vi "Detect Failed.vi"(8 "error in (no error)":errorcluster, 9 "Software-Only?":bool, 10 "Targets in":T1 {"Filtered Targets"."IP Mode" items=["Static"=1, "DHCP/Link-Local"=2, "Link-Local Only"=4, "DHCP Only"=8]}, 11 "Ctl Refs in":T5) -> (0 "error out":errorcluster, 1 "Enum":T4, 2 "Targets out":T1 {"Filtered Targets"."IP Mode" items=["Static"=1, "DHCP/Link-Local"=2, "Link-Local Only"=4, "DHCP Only"=8]}, 3 "Ctl Refs out":T5)   [LabVIEW 2013]
uses:
  Controls/Refs.ctl
  Controls/Button Refs.ctl
  Controls/Tab Ctl Refs.ctl
  types/TabStateType.ctl
  Controls/Indicator Refs.ctl
  Controls/Slider Refs.ctl
  Controls/Control Refs.ctl
  types/ButtonStateType.ctl
  Controls/Targets.ctl
  Controls/Detected.ctl
  types/MAX Sys Cfg Target Information.ctl
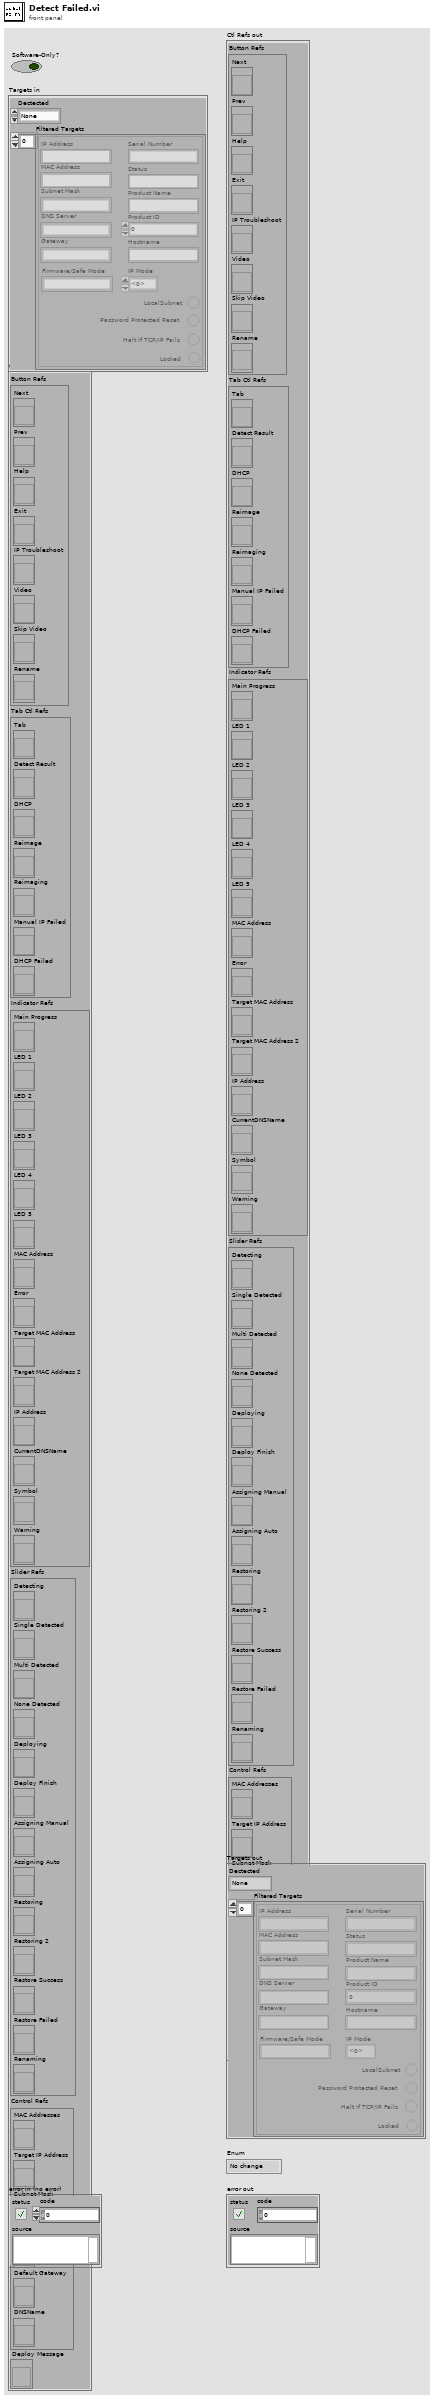
[diagram p1: front panel]
types:
  T1 = typedef "Targets.ctl" = cluster{"Dectected":T2, "Filtered Targets":T3[]}
  T2 = typedef "Detected.ctl" = enum16{"None", "Failed", "Single", "Multi"}
  T3 = typedef "MAX Sys Cfg Target Information.ctl" = cluster{"MAC Address":string, "IP Address":string, "Status":string, "Product Name":string, "Hostname":string, "Firmware/Safe Mode":string, "Subnet Mask":string, "Gateway":string, "DNS Server":string, "Serial Number":string, "Product ID":u32, "Locked ":bool, "LocalSubnet":bool, "Halt If TCP/IP Fails":bool, "Password Protected Reset":bool, "IP Mode":i32}
  T4 = typedef "ButtonStateType.ctl" = enum16{"No change", "No Next", "No Prev", "All Disabled", "All Enabled", "Exit Only"}
  T5 = typedef "Refs.ctl" = cluster{"Button Refs":T6, "Tab Ctl Refs":T7, "Indicator Refs":T8, "Slider Refs":T9, "Control Refs":T10, "Deploy Message":refnum<vi>}
  T6 = typedef "Button Refs.ctl" = cluster{"Next":refnum<vi>, "Prev":refnum<vi>, "Help":refnum<vi>, "Exit":refnum<vi>, "IP Troubleshoot":refnum<vi>, "Video":refnum<vi>, "Skip Video":refnum<vi>, "Rename":refnum<vi>}
  T7 = typedef "Tab Ctl Refs.ctl" = cluster{"Tab":refnum<vi>, "Detect Result":refnum<vi>, "DHCP":refnum<vi>, "Reimage":refnum<vi>, "Reimaging":refnum<vi>, "Manual IP Failed":refnum<vi>, "DHCP Failed":refnum<vi>}
  T8 = typedef "Indicator Refs.ctl" = cluster{"Main Progress":refnum<vi>, "LED 1":refnum<vi>, "LED 2":refnum<vi>, "LED 3":refnum<vi>, "LED 4":refnum<vi>, "LED 5":refnum<vi>, "MAC Address":refnum<vi>, "Error":refnum<vi>, "Target MAC Address":refnum<vi>, "Target MAC Address 2":refnum<vi>, "IP Address":refnum<vi>, "CurrentDNSName":refnum<vi>, "Symbol":refnum<vi>, "Warning":refnum<vi>}
  T9 = typedef "Slider Refs.ctl" = cluster{"Detecting":refnum<vi>, "Single Detected":refnum<vi>, "Multi Detected":refnum<vi>, "None Detected":refnum<vi>, "Deploying":refnum<vi>, "Deploy Finish":refnum<vi>, "Assigning Manual":refnum<vi>, "Assigning Auto":refnum<vi>, "Restoring":refnum<vi>, "Restoring 2":refnum<vi>, "Restore Success":refnum<vi>, "Restore Failed":refnum<vi>, "Renaming":refnum<vi>}
  T10 = typedef "Control Refs.ctl" = cluster{"MAC Addresses":refnum<vi>, "Target IP Address":refnum<vi>, "Subnet Mask":refnum<vi>, "DNS IP":refnum<vi>, "Default Gateway":refnum<vi>, "DNSName":refnum<vi>}
  T11 = enum32{"Welcome", "Instructions", "Detect", "Run Detection", "Detect Result", "Deploy", "Run Deployment", "Connect Verify", "Success"}
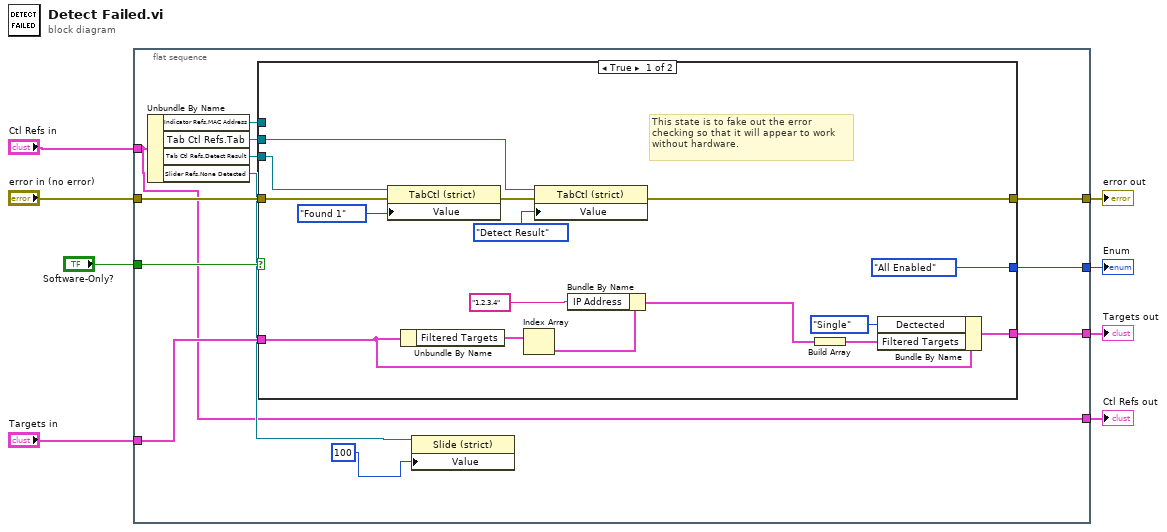
[diagram p0: block diagram]
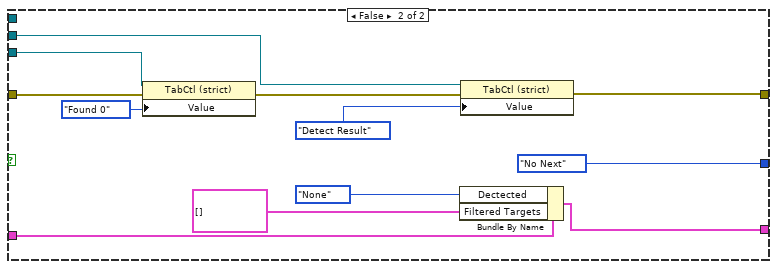
[diagram p2: hidden frame]
diagram:
  n1 = flat-sequence {
    tunnel: "error in (no error)" -> [w20]
    tunnel: [w19] -> w2
    tunnel: "Targets in" -> [w18]
    tunnel: [w17] -> w4
    tunnel: "Software-Only?" -> [w16]
    tunnel: [w15] -> w6
    tunnel: "Ctl Refs in" -> [w10]
    tunnel: [w10] -> w8
    frame #0 {
      n2 = Unbundle By Name(w10) -> ("Indicator Refs.MAC Address"=w9:refnum<vi>, "Tab Ctl Refs.Tab"=w13:refnum<vi>, "Tab Ctl Refs.Detect Result"=w14:refnum<vi>, "Slider Refs.None Detected"=w11:refnum<vi>)
      n3 = case shown="True" w16 {
        tunnel: w20 -> [w35 w47]
        tunnel: [w32 w44] -> w19
        tunnel: w18 -> [w26 w42]
        tunnel: [w23 w39] -> w17
        tunnel: [ButtonStateType."All Enabled" ("Enum") ButtonStateType."No Next" ("Enum")] -> w15
        tunnel: w14 -> [w22 w38]
        tunnel: w13 -> [w21 w37]
        tunnel: w9 -> [_ _]
        frame True {
          # "This state is to fake out the error\nchecking so that it will appear to work\nwithout hardware."
          n4 = property on="Property Node" class="TabCtl (strict)"(reference=w22, error in=w35, "Value"=enum32{"Found 0", "Found 1", "Found 2"}."Found 1" ("Detect Result Tabs")) -> (error out=w34:errorcluster)  [unwired: 1 out]
          n5 = Unbundle By Name(w26) -> ("Filtered Targets"=w27:T3[])
          n6 = Index Array(array=w27) -> (element=w30:T3)  [unwired: 1 in]
          n7 = property on="Property Node" class="TabCtl (strict)"(reference=w21, error in=w34, "Value"=T11."Detect Result" ("Tab Control")) -> (error out=w32:errorcluster)  [unwired: 1 out]
          n8 = Bundle By Name(cluster=w30, "IP Address"="1.2.3.4") -> (w31:T3)
          n9 = Build Array(w31) -> (w24:T3[])
          n10 = Bundle By Name(cluster=w26, "Dectected"=Detected."Single", "Filtered Targets"=w24) -> (w23:T1)
        }
        frame False {
          n11 = property on="Property Node" class="TabCtl (strict)"(reference=w38, error in=w47, "Value"=enum32{"Found 0", "Found 1", "Found 2"}."Found 0" ("Detect Result Tabs")) -> (error out=w46:errorcluster)  [unwired: 1 out]
          n12 = Bundle By Name(cluster=w42, "Dectected"=Detected."None", "Filtered Targets"=T3[] []) -> (w39:T1)
          n13 = property on="Property Node" class="TabCtl (strict)"(reference=w37, error in=w46, "Value"=T11."Detect Result" ("Tab Control")) -> (error out=w44:errorcluster)  [unwired: 1 out]
        }
      }
      n14 = property on="Property Node" class="Slide (strict)"(reference=w11, "Value"=i8 100 ("Slide 5")) -> ()  [unwired: 1 in, 2 out]
    }
  }
  "Ctl Refs out" <- w8
  "Enum" <- w6
  "Targets out" <- w4
  "error out" <- w2
